vi "updateCamera.vi"(8 "error in (no error)":errorcluster, 10 "data":T1, 11 "AtomChipHWC in":refnum<class "AtomChipHWC.lvclass">) -> (0 "error out":errorcluster, 3 "AtomChipHWC out":refnum<class "AtomChipHWC.lvclass">)   [LabVIEW 2009, in "Hardware.lvlib" / "HWControllers.lvlib" / "AtomChipHWC.lvclass"]
uses:
  AtomChipHWC.lvclass
panel:
  # "start - stop in type?"
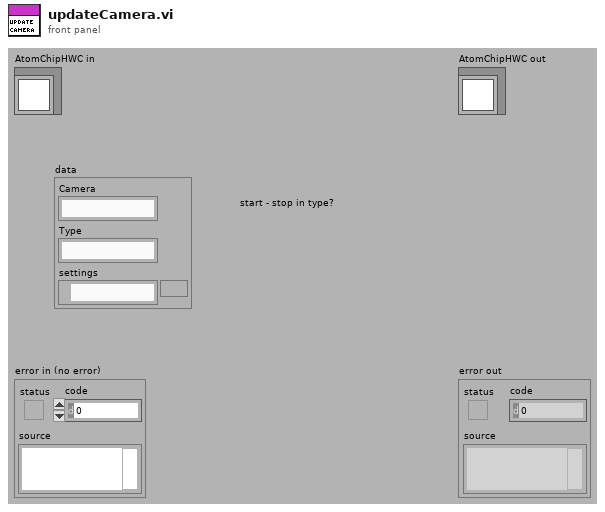
[diagram p1: front panel]
types:
  T1 = cluster{"Camera":string, "Type":string, "settings":path}
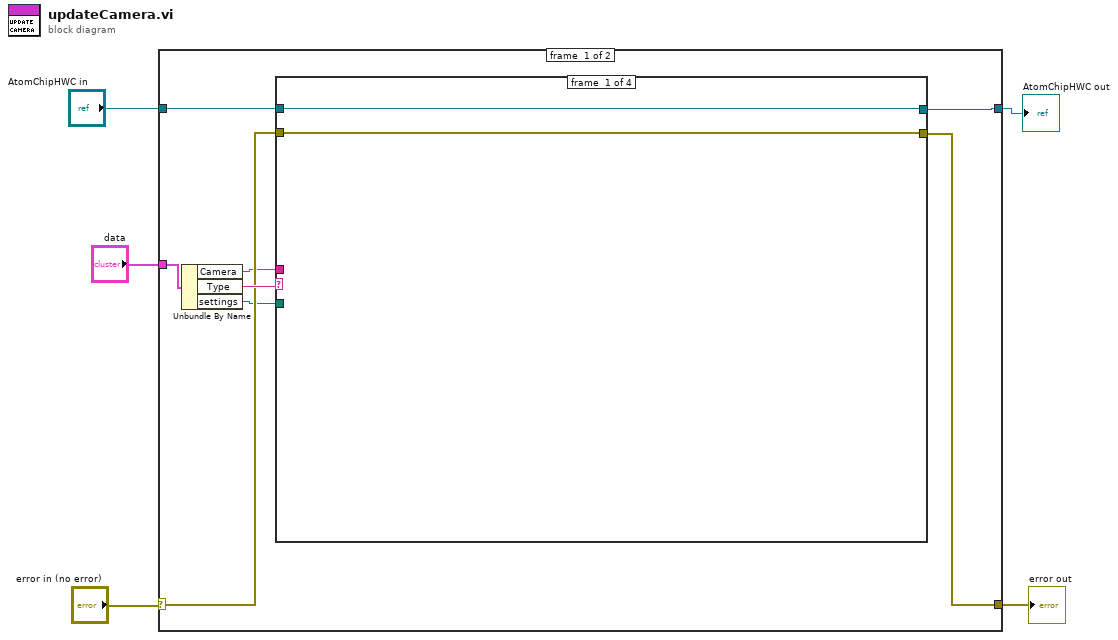
[diagram p0: block diagram]
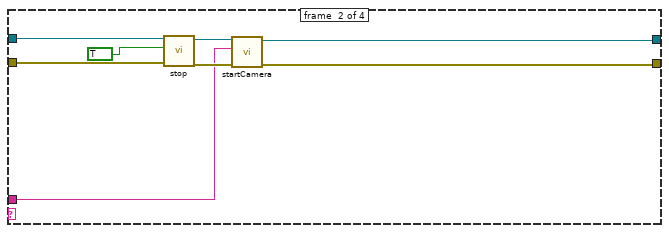
[diagram p2: hidden frame]
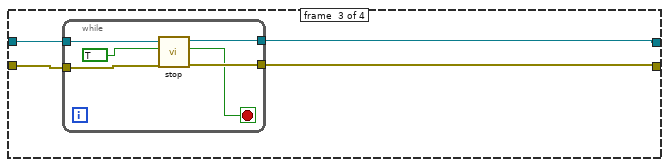
[diagram p3: hidden frame]
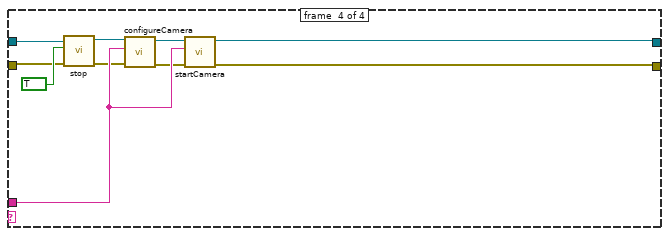
[diagram p4: hidden frame]
diagram:
  n1 = case shown="No Error" "error in (no error)" {
    selector: "error in (no error)" -> [w10 w44]
    tunnel: [w9 w45] -> w4
    tunnel: "AtomChipHWC in" -> [w11 w45]
    tunnel: [w8 w44] -> w2
    tunnel: "data" -> [w13 _]
    frame #0 {
      n2 = Unbundle By Name(w13) -> ("Camera"=w6:string, "Type"=w12:string, "settings"=w7:path)
      n3 = case shown="\"start\"" w12 {
        tunnel: w11 -> [w15 w22 w27 w37]
        tunnel: w10 -> [w14 w21 w25 w34]
        tunnel: [w15 w18 w26 w40] -> w9
        tunnel: [w14 w17 w24 w39] -> w8
        tunnel: w7 -> [_ _ _ _]
        tunnel: w6 -> [_ w16 _ w42]
        frame #0 {
        }
        frame #1 {
          n4 = call-dynamic "stop.vi"("error in (no error)"=w21, "stop?"=TRUE, "AtomChipHWC in"=w22) -> ("error out"=w19:errorcluster, "AtomChipHWC out"=w20:refnum<class "AtomChipHWC.lvclass">)  [unwired: 6 in, 1 out]
          n5 = call "startCamera.vi"("error in (no error)"=w19, "camera"=w16, "AtomChipHWC in"=w20) -> ("error out"=w17:errorcluster, "AtomChipHWC out"=w18:refnum<class "AtomChipHWC.lvclass">)  [unwired: 7 in]
        }
        frame #2 {
          n6 = while {
            tunnel: w27 -> [w32]
            tunnel: [w31] -> w26
            tunnel: w25 -> [w30]
            tunnel: [w29] -> w24
            stop <- w28 stop-if-true
            n7 = call-dynamic "stop.vi"("error in (no error)"=w30, "stop?"=TRUE, "AtomChipHWC in"=w32) -> ("error out"=w29:errorcluster, "stopped"=w28:bool, "AtomChipHWC out"=w31:refnum<class "AtomChipHWC.lvclass">)  [unwired: 6 in]
          }
        }
        frame #3 {
          n8 = call-dynamic "stop.vi"("error in (no error)"=w34, "stop?"=TRUE, "AtomChipHWC in"=w37) -> ("error out"=w35:errorcluster, "AtomChipHWC out"=w36:refnum<class "AtomChipHWC.lvclass">)  [unwired: 6 in, 1 out]
          n9 = call "configureCamera.vi"("error in (no error)"=w35, "device"=w42, "AtomChipHWC in"=w36) -> ("error out"=w41:errorcluster, "AtomChipHWC out"=w43:refnum<class "AtomChipHWC.lvclass">)  [unwired: 7 in]
          n10 = call "startCamera.vi"("error in (no error)"=w41, "camera"=w42, "AtomChipHWC in"=w43) -> ("error out"=w39:errorcluster, "AtomChipHWC out"=w40:refnum<class "AtomChipHWC.lvclass">)  [unwired: 7 in]
        }
      }
    }
    frame #1 {
    }
  }
  "error out" <- w2
  "AtomChipHWC out" <- w4
